vi "Global PREDCIR.vi"() -> ()   [LabVIEW 2020]
panel:
  out "PREDCIR":T1
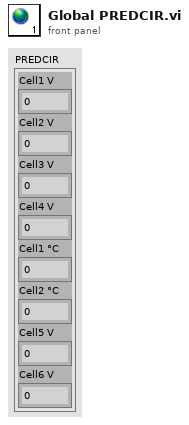
[diagram p1: front panel]
types:
  T1 = cluster{"Cell1 V":sgl, "Cell2 V":sgl, "Cell3 V":sgl, "Cell4 V":sgl, "Cell1 °C":sgl, "Cell2 °C":sgl, "Cell5 V":sgl, "Cell6 V":sgl}
diagram:
